vi "PH_IEEE1394Camera.ProcPeriodic.vi"(0 "i ref in":refnum<vi>, 3 "ms timeout (100)":i32=100, 5 "error in (no error)":errorcluster) -> (14 "i ref out":refnum<vi>, 17 "timed out":bool, 19 "error out":errorcluster)   [LabVIEW 2014, in "PH_IEEE1394Camera.lvlib"]
doc: "This method serves to periodically do things like reading values from the HW. Methods that should be executed periodically should be called from THIS methode. Add code here."
uses:
  PH_IEEE1394Camera.lvlib
  PH_Basics/PH_StatusHandler/PH_StatusHandler.Status.ctl
  PH_Basics/PH_Cam_BaseClass/PH_Cam_BaseClass.lvlib
  <vilib>/vision/driver/NI_Vision_Acquisition_Software.lvlib
  CS_Core/BaseProcess/BaseProcess.lvlib
  PH_Basics/PH_StatusHandler/PH_StatusHandler.lvlib
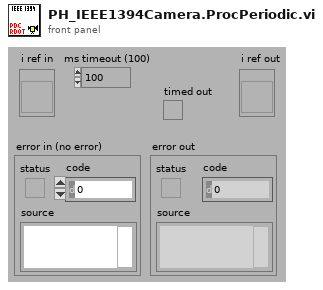
[diagram p1: front panel]
types:
  T1 = typedef "PH_Cam_BaseClass.lvlib/PH_Cam_BaseClass.i attribute.ctl" = cluster{"Gui Refs":T2, "Cam":cluster{"Source Notifier":refnum<notifier>, "Error":errorcluster, "Camera ID":string}, "Images":cluster{"Cam":T3, "Operation":T3, "PSDB":T3}, "Window Image":cluster{"Indicate Image":bool, "Window No.":i32, "Scale Facor":dbl, "Center Cross":bool, "Subtract Backgr":bool, "CoG":bool, "Color Palette":cluster{"Red":u8, "Green":u8, "Blue":u8}[], "Image On":bool}, "Default Prdc Int":i32, "Performance":cluster{"on":bool, "Timestamp Last Frame":i32}, "Histogram":cluster{"on":bool, "Mapping":bool}, "Save Image":cluster{"Save":bool, "File refnum":refnum<file>}, "Setting Service ID":i32, "Screen":cluster{"x-resolution":i16, "y-resolution":i16}, "On":bool, "Constructor finished":bool, "configured":bool}
  T2 = typedef "PH_Cam_BaseClass.lvlib/PH_Cam_BaseClass.GUI Refs.ctl" = cluster{"Frame Rate":refnum<vi>, "Get Frame Rate":refnum<vi>, "Show Image":refnum<vi>, "Get Histogram":refnum<vi>, "Mapping":refnum<vi>, "Histogram":refnum<vi>, "Center Cross":refnum<vi>, "Center of Gravity":refnum<vi>, "Scale Factor [%]":refnum<vi>, "Save Image":refnum<vi>, "Palette":refnum<vi>, "Subtract Background":refnum<vi>, "Cam Error":refnum<vi>, "On":refnum<vi>, "Cam List":refnum<vi>}
  T3 = typedef "IMAQ Image.ctl" = refnum<image>
  T4 = typedef "PH_StatusHandler.lvlib/PH_StatusHandler.Status.ctl" = i16
  T5 = typedef "PH_IEEE1394Camera.lvlib/PH_IEEE1394Camera.i attribute.ctl" = cluster{"Gui Refs":cluster{"Brightness":refnum<vi>, "Shutter":refnum<vi>, "Gain":refnum<vi>, "Center of Gravity":refnum<vi>, "Supported Video Modes":refnum<vi>, "Trigger Polarity":refnum<vi>, "Trigger Mode":refnum<vi>, "Trigger Timeout":refnum<vi>, "Bit Depth":refnum<vi>, "Video Mode":refnum<vi>, "Top":refnum<vi>, "Bottom":refnum<vi>, "Left":refnum<vi>, "Right":refnum<vi>, "Set ROI to Maximum":refnum<vi>, "Camera Details":refnum<vi>, "Current Cam Attributes":refnum<vi>, "Attribute to set":refnum<vi>, "Num Value":refnum<vi>, "String Value":refnum<vi>, "Bool Value":refnum<vi>, "Set Cam Attribute":refnum<vi>}, "Cam":cluster{"IMAQ1394 Session":T6, "Camera Details":T7}, "Current Attributes":T8[], "Supported Video Modes ":cluster{"Video Mode":u32, "Video Mode Name":string}[], "Wanted Attributes":cluster{"Name":string, "Num Value":dbl, "String Value":string, "Boolean Value":bool}[], "Cam Attributes":T10}
  T6 = typedef "IMAQdx.ctl" = refnum<k21>
  T7 = typedef "PH_IEEE1394Camera.lvlib/PH_IEEE1394Camera.Cam Details.ctl" = cluster{"Model":string, "Serial Number":dbl, "Cam name (Machinery)":string, "Bus Type":string}
  T8 = typedef "PH_IEEE1394Camera.lvlib/PH_IEEE1394Camera.Cam Attribute.ctl" = cluster{"Information":cluster{"Type":T9, "Readable":bool, "Writable":bool, "Name":string}, "Num Value":dbl, "String Value":string, "Maximum":dbl, "Minimum":dbl, "Units":string, "Description":string, "EnumStrings[]":string[], "EnumValues[]":u32[], "Boolean Value":bool}
  T9 = typedef "NI_Vision_Acquisition_Software.lvlib/IMAQdx Attribute Type.ctl" = enum32{"U32", "I64", "DBL", "String", "Enum", "Bool", "Command"}
  T10 = typedef "PH_IEEE1394Camera.lvlib/PH_IEEE1394Camera.Relevant Cam Attributes.ctl" = cluster{"Video Mode":cluster{"Name":string, "Index":i32}, "Brightness":cluster{"Name":string, "Index":i32}, "Gain":cluster{"Name":string, "Index":i32}, "Shutter":cluster{"Name":string, "Index":i32}, "Trigger Pol":cluster{"Name":string, "Index":i32}, "Trigger Mode":cluster{"Name":string, "Index":i32}, "Timeout":cluster{"Name":string, "Index":i32}, "Bit Depth":cluster{"Name":string, "Index":i32}, "Pixel Bits":cluster{"Name":string, "Index":i32}, "Pixel Bytes":cluster{"Name":string, "Index":i32}, "Left":cluster{"Name":string, "Index":i32}, "Right":cluster{"Name":string, "Index":i32}, "Top":cluster{"Name":string, "Index":i32}, "Bottom":cluster{"Name":string, "Index":i32}}
  T11 = typedef "PH_Cam_BaseClass.lvlib/PH_Cam_BaseClass.Settings.ctl" = cluster{"Cam ID":string, "Gain":dbl, "Brightness":dbl, "Shutter":dbl, "Mode":i32}
  T12 = cluster{"Name":string, "Num Value":dbl, "String Value":string, "Boolean Value":bool}[]
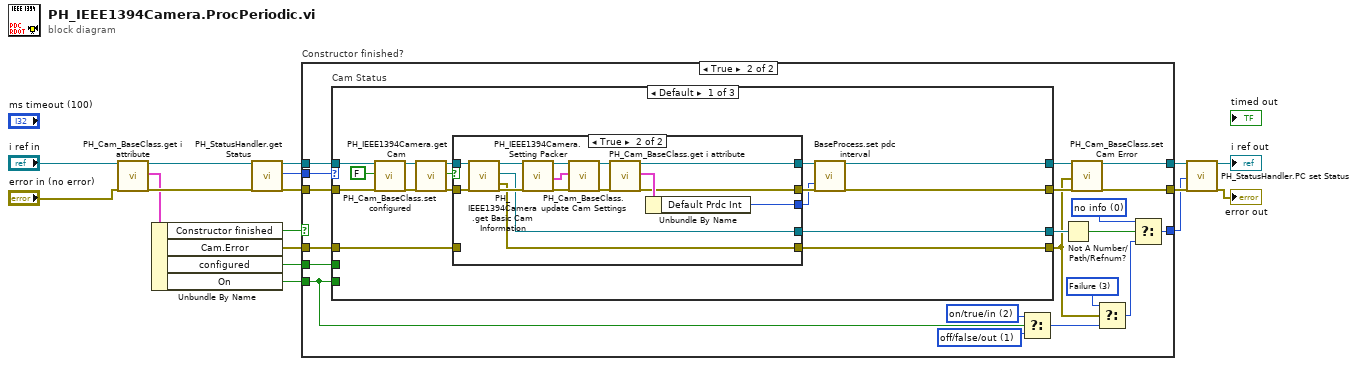
[diagram p0: block diagram]
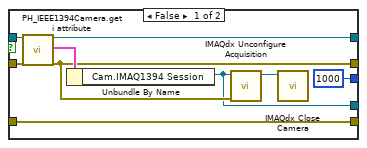
[diagram p3: hidden frame]
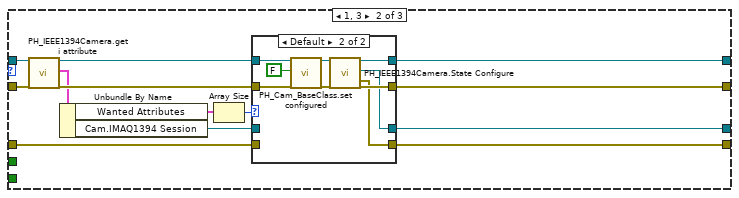
[diagram p4: hidden frame]
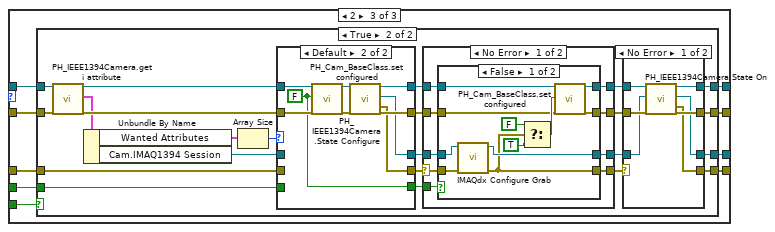
[diagram p6: hidden frame]
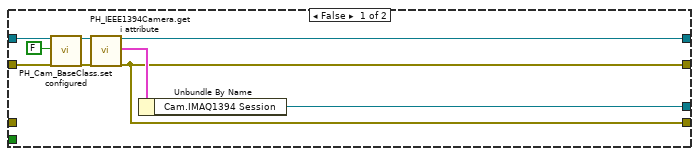
[diagram p7: hidden frame]
diagram:
  n1 = call "PH_Cam_BaseClass.get i attribute.vi"("i ref in"="i ref in", "error in (no error)"="error in (no error)") -> ("i ref out"=w2:refnum<vi>, "i attribute"=w14:T1, "error out"=w16:errorcluster)  [unwired: 15 in]
  n2 = Unbundle By Name(w14) -> ("Constructor finished"=w13:bool, "Cam.Error"=w12:errorcluster, "configured"=w5:bool, "On"=w7:bool)
  n3 = call "PH_StatusHandler.get Status.vi"("VI in"=w2, "error in"=w16) -> ("VI out"=w1:refnum<vi>, "Status"=w3:T4, "error out"=w4:errorcluster)  [unwired: 15 in]
  n4 = case "Constructor finished?" shown="True" w13 {
    tunnel: [w20 w36] -> w8
    tunnel: [w19 w35] -> w10
    tunnel: w4 -> [w19 w40]
    tunnel: w1 -> [w20 w39]
    tunnel: w3 -> [w18 w38]
    tunnel: w12 -> [_ w37]
    tunnel: w7 -> [_ w22]
    tunnel: [w18 w23] -> w6
    tunnel: w5 -> [_ w21]
    frame False {
    }
    frame True {
      w27 = T4 1 items=["no info", "off/false/out", "on/true/in", "Failure", "Alarm", "Status 1", "Status 2", "Status 3"] ("Cam State")
      w28 = T4 2 items=["no info", "off/false/out", "on/true/in", "Failure", "Alarm", "Status 1", "Status 2", "Status 3"] ("Cam State")
      w29 = T4 3 items=["no info", "off/false/out", "on/true/in", "Failure", "Alarm", "Status 1", "Status 2", "Status 3"] ("Cam State")
      w30 = T4 0 items=["no info", "off/false/out", "on/true/in", "Failure", "Alarm", "Status 1", "Status 2", "Status 3"] ("Cam State")
      n5 = case "Cam Status" shown="Default" w38 {
        tunnel: [w51 w93 w115] -> w32
        tunnel: [w53 w92 w114] -> w31
        tunnel: w40 -> [w46 w91 w113]
        tunnel: w39 -> [w44 w89 w112]
        tunnel: [w48 w81 w111] -> w24
        tunnel: w37 -> [w41 w84 w108]
        tunnel: [w47 w82 w109] -> w26
        tunnel: w22 -> [_ _ w110]
        tunnel: w21 -> [_ _ w107]
        frame Default {
          n6 = call "PH_Cam_BaseClass.set configured.vi"("i ref in"=w44, "configured"=FALSE, "error in (no error)"=w46) -> ("i ref out"=w43:refnum<vi>, "error out"=w45:errorcluster)  [unwired: 15 in]
          n7 = call "PH_IEEE1394Camera.get Cam.vi"("i ref in"=w43, "error in"=w45) -> ("i ref out"=w56:refnum<vi>, "Cam found"=w54:bool, "error out"=w55:errorcluster)  [unwired: 14 in, 1 out]
          n8 = case shown="True" w54 {
            tunnel: w56 -> [w60 w80]
            tunnel: w55 -> [w59 w79]
            tunnel: [w61 w72] -> w50
            tunnel: [w58 w68] -> w52
            tunnel: [1000 ("Default Prdc Int") w71] -> w49
            tunnel: [w64 w66] -> w48
            tunnel: w41 -> [w64 _]
            tunnel: [w57 w67] -> w47
            frame False {
              n9 = call "PH_IEEE1394Camera.get i attribute.vi"("i ref in"=w60, "error in (no error)"=w59) -> ("i ref out"=w61:refnum<vi>, "i attribute"=w63:T5, "error out"=w58:errorcluster)  [unwired: 15 in]
              n10 = Unbundle By Name(w63) -> ("Cam.IMAQ1394 Session"=w57:T6)
              n11 = call <vilib>:"IMAQdx Unconfigure Acquisition.vi"("error in"=w58, "Session In"=w57) -> ("Session Out"=w62:T6)  [unwired: 8 in, 1 out]
              n12 = call <vilib>:"IMAQdx Close Camera.vi"("Session In"=w62) -> ()  [unwired: 10 in, 1 out]
            }
            frame True {
              n13 = call "PH_IEEE1394Camera.get Basic Cam Information.vi"("i ref in"=w80, "error in (no error)"=w79) -> ("i ref out"=w78:refnum<vi>, "IMAQ1394 Session Out"=w67:T6, "Cam Error out"=w66:errorcluster, "error out"=w76:errorcluster)  [unwired: 14 in]
              n14 = call "PH_IEEE1394Camera.Setting Packer.vi"("i ref in"=w78, "error in (no error)"=w76) -> ("i ref out"=w77:refnum<vi>, "Cam Settings"=w74:T11, "error out"=w75:errorcluster)  [unwired: 15 in]
              n15 = call "PH_Cam_BaseClass.update Cam Settings.vi"("VI in"=w77, "Cam Settings In"=w74, "error in (no error)"=w75) -> ("VI out"=w73:refnum<vi>, "error out"=w69:errorcluster)  [unwired: 15 in]
              n16 = call "PH_Cam_BaseClass.get i attribute.vi"("i ref in"=w73, "error in (no error)"=w69) -> ("i ref out"=w72:refnum<vi>, "i attribute"=w70:T1, "error out"=w68:errorcluster)  [unwired: 15 in]
              n17 = Unbundle By Name(w70) -> ("Default Prdc Int"=w71:i32)
            }
          }
          n18 = call "BaseProcess.set pdc interval.vi"("i ref in"=w50, "PeriodicInterval [ms]"=w49, "error in (no error)"=w52) -> ("i ref out"=w51:refnum<vi>, "error out"=w53:errorcluster)  [unwired: 14 in, 1 out]
        }
        frame 1, 3 {
          n19 = call "PH_IEEE1394Camera.get i attribute.vi"("i ref in"=w89, "error in (no error)"=w91) -> ("i ref out"=w88:refnum<vi>, "i attribute"=w87:T5, "error out"=w90:errorcluster)  [unwired: 15 in]
          n20 = Unbundle By Name(w87) -> ("Wanted Attributes"=w86:T12, "Cam.IMAQ1394 Session"=w83:T6)
          n21 = Array Size(array=w86) -> (size(s)=w85:i32)
          n22 = case shown="Default" w85 {
            tunnel: [w97 w106] -> w93
            tunnel: [w96 w105] -> w92
            tunnel: [w95 w102] -> w81
            tunnel: w90 -> [w96 w104]
            tunnel: w88 -> [w97 w100]
            tunnel: w84 -> [w95 _]
            tunnel: [w94 w103] -> w82
            tunnel: w83 -> [w94 _]
            frame 0 {
            }
            frame Default {
              n23 = call "PH_Cam_BaseClass.set configured.vi"("i ref in"=w100, "configured"=FALSE, "error in (no error)"=w104) -> ("i ref out"=w99:refnum<vi>, "error out"=w101:errorcluster)  [unwired: 15 in]
              n24 = call "PH_IEEE1394Camera.State Configure.vi"("VI in"=w99, "error in (no error)"=w101) -> ("VI out"=w106:refnum<vi>, "Session Out"=w103:T6, "Cam Error"=w102:errorcluster, "error out"=w105:errorcluster)  [unwired: 14 in]
            }
          }
        }
        frame 2 {
          n25 = case shown="True" w110 {
            tunnel: [w117 w147] -> w115
            tunnel: [w116 w146] -> w114
            tunnel: w113 -> [w121 w137]
            tunnel: w112 -> [w119 w136]
            tunnel: [w116 w144] -> w111
            tunnel: [w123 w145] -> w109
            tunnel: w108 -> [_ w135]
            tunnel: w107 -> [_ w127]
            frame False {
              n26 = call "PH_Cam_BaseClass.set configured.vi"("i ref in"=w119, "configured"=FALSE, "error in (no error)"=w121) -> ("i ref out"=w118:refnum<vi>, "error out"=w122:errorcluster)  [unwired: 15 in]
              n27 = call "PH_IEEE1394Camera.get i attribute.vi"("i ref in"=w118, "error in (no error)"=w122) -> ("i ref out"=w117:refnum<vi>, "i attribute"=w124:T5, "error out"=w116:errorcluster)  [unwired: 15 in]
              n28 = Unbundle By Name(w124) -> ("Cam.IMAQ1394 Session"=w123:T6)
            }
            frame True {
              n29 = call "PH_IEEE1394Camera.get i attribute.vi"("i ref in"=w136, "error in (no error)"=w137) -> ("i ref out"=w142:refnum<vi>, "i attribute"=w141:T5, "error out"=w143:errorcluster)  [unwired: 15 in]
              n30 = Unbundle By Name(w141) -> ("Wanted Attributes"=w140:T12, "Cam.IMAQ1394 Session"=w138:T6)
              n31 = Array Size(array=w140) -> (size(s)=w139:i32)
              n32 = case shown="Default" w139 {
                tunnel: [w191 w200] -> w128
                tunnel: [w190 w199] -> w130
                tunnel: [w189 w196] -> w126
                tunnel: w143 -> [w190 w198]
                tunnel: w142 -> [w191 w194]
                tunnel: w135 -> [w189 _]
                tunnel: [w188 w197] -> w133
                tunnel: w138 -> [w188 _]
                tunnel: [w187 w192] -> w125
                tunnel: w127 -> [w187 _]
                frame 0 {
                }
                frame Default {
                  w192 = FALSE ("configured")
                  n33 = call "PH_Cam_BaseClass.set configured.vi"("i ref in"=w194, "configured"=w192, "error in (no error)"=w198) -> ("i ref out"=w193:refnum<vi>, "error out"=w195:errorcluster)  [unwired: 15 in]
                  n34 = call "PH_IEEE1394Camera.State Configure.vi"("VI in"=w193, "error in (no error)"=w195) -> ("VI out"=w200:refnum<vi>, "Session Out"=w197:T6, "Cam Error"=w196:errorcluster, "error out"=w199:errorcluster)  [unwired: 14 in]
                }
              }
              n35 = case shown="No Error" w126 {
                selector: w126 -> [w150 w173]
                tunnel: [w156 w172] -> w134
                tunnel: w133 -> [w155 w172]
                tunnel: [w149 w173] -> w132
                tunnel: [w154 w174] -> w131
                tunnel: w130 -> [w153 w174]
                tunnel: [w152 w175] -> w129
                tunnel: w128 -> [w151 w175]
                tunnel: w125 -> [w148 _]
                frame No Error {
                  n36 = case shown="False" w148 {
                    tunnel: [w160 w169] -> w156
                    tunnel: w155 -> [w162 w169]
                    tunnel: [w158 w170] -> w154
                    tunnel: w153 -> [w163 w170]
                    tunnel: [w157 w171] -> w152
                    tunnel: w151 -> [w164 w171]
                    tunnel: w150 -> [w161 w168]
                    tunnel: [w159 w168] -> w149
                    frame False {
                      n37 = call <vilib>:"IMAQdx Configure Grab.vi"("error in"=w161, "Session In"=w162) -> ("error out"=w159:errorcluster, "Session Out"=w160:T6)  [unwired: 8 in]
                      n38 = Select(t=FALSE, s=w159, f=TRUE ("configured")) -> (s? t:f=w165:bool)
                      n39 = call "PH_Cam_BaseClass.set configured.vi"("i ref in"=w164, "configured"=w165, "error in (no error)"=w163) -> ("i ref out"=w157:refnum<vi>, "error out"=w158:errorcluster)  [unwired: 15 in]
                    }
                    frame True {
                    }
                  }
                }
                frame Error {
                }
              }
              n40 = case shown="No Error" w132 {
                selector: w132 -> [_ w183]
                tunnel: [w182 w186] -> w147
                tunnel: [w181 w185] -> w146
                tunnel: [w180 w184] -> w145
                tunnel: [w179 w183] -> w144
                tunnel: w131 -> [w178 w185]
                tunnel: w129 -> [w177 w186]
                tunnel: w134 -> [w176 w184]
                frame No Error {
                  n41 = call "PH_IEEE1394Camera.State On.vi"("VI in"=w177, "IMAQ1394 Session in"=w176, "error in (no error)"=w178) -> ("VI out"=w182:refnum<vi>, "IMAQ1394 Session out"=w180:T6, "Cam Error"=w179:errorcluster, "error out"=w181:errorcluster)  [unwired: 13 in]
                }
                frame Error {
                }
              }
            }
          }
        }
      }
      n42 = Select(t=w28, s=w22, f=w27) -> (s? t:f=w25:T4)
      n43 = Not A Number/Path/Refnum?(number/path/refnum=w26) -> (NaN/Path/Refnum?=w34:bool)
      n44 = call "PH_Cam_BaseClass.set Cam Error.vi"("VI in"=w32, "Cam Error"=w24, "error in"=w31) -> ("VI out"=w36:refnum<vi>, "error out"=w35:errorcluster)  [unwired: 15 in]
      n45 = Select(t=w29, s=w24, f=w25) -> (s? t:f=w33:T4)
      n46 = Select(t=w30, s=w34, f=w33) -> (s? t:f=w23:T4)
    }
  }
  n47 = call "PH_StatusHandler.PC set Status.vi"("i ref in"=w8, "Status"=w6, "error in (no error)"=w10) -> ("i ref out"=→"i ref out":refnum<vi>, "error out"=→"error out":errorcluster)  [unwired: 15 in]
